vi "kvCanIoCtlSet.vi"(2 "error in (no error)":errorcluster, 3 "Function":T1(ring), 4 "Channel Handle (input only)":i32) -> (0 "error out":errorcluster, 1 "Channel Handle (ouput only)":i32)   [LabVIEW 2022 SP3]
doc: "Performs I/O Control \"set\" functions:\n\nItem \"Prefer Extended Ids\": Tells CANLIB to \"prefer\" extended identifiers; that is, if you send a message with canWrite() and don't specify canMSG_EXT nor canMSG_STD, canMSG_EXT will be assumed. canRead() et al will set canMSG_EXT and/or canMSG_STD as usual and are not affected by this call. \n\nItem \"Prefer Standard Ids\": Tells CANLIB to \"prefer\" standard identifiers; that is, if you send a message with canWrite() and don't specify canMSG_EXT nor canMSG_STD, canMSG_STD will be assumed. canRead() et al will set canMSG_EXT and/or canMSG_STD as usual and are not affected by this call. \n\nItem \"Clear Error Counters\": Tells CANLIB to clear the CAN error counters. Note that not all CAN controllers support this operation."
uses:
  canlib32.dll
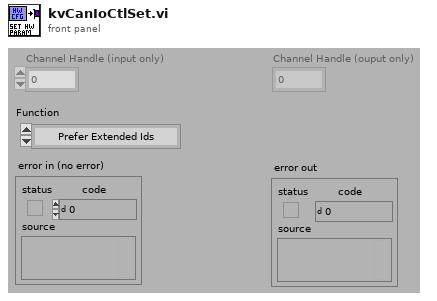
[diagram p1: front panel]
types:
  T1 = enum16{"Prefer Extended Ids", "Prefer Standard Ids", "Clear Error Counters"}
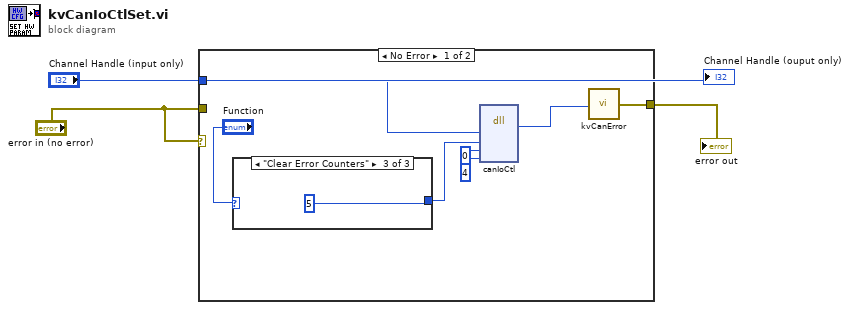
[diagram p0: block diagram]
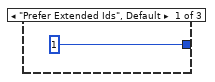
[diagram p2: hidden frame]
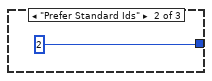
[diagram p3: hidden frame]
diagram:
  n1 = case shown="No Error" "error in (no error)" {
    tunnel: [w10 w14] -> w3
    tunnel: "error in (no error)" -> [_ w14]
    tunnel: "Channel Handle (input only)" -> [w8 _]
    frame No Error {
      n2 = case shown="\"Clear Error Counters\"" "Function" {
        tunnel: [1 2 5] -> w4
        frame "Prefer Extended Ids", Default {
        }
        frame "Prefer Standard Ids" {
        }
        frame "Clear Error Counters" {
        }
      }
      n3 = dll-call lib="canlib32.dll" fn="canIoCtl" label="Call canIoCtl"("handle"=w8, "func"=w4, "buf"=0, "buflen"=4) -> (w9:i32)  [unwired: 7 in, 2 out]
      n4 = call "kvCanError.vi"("error code"=w9) -> ("error out"=w10:errorcluster)
    }
    frame Error {
    }
  }
  "error out" <- w3
  "Channel Handle (ouput only)" <- "Channel Handle (input only)"
